vi "PmuPktDecode.vi"(8 "error in (no error)":errorcluster, 10 "PktData":string) -> (0 "error out":errorcluster, 1 "MsgVersion":u8, 2 "PMUDataType":T1, 3 "PktData":u8[](array[numeric]) format="%x", 5 "SyncOK":bool)   [LabVIEW 2014, in "SensorPlugins.lvlib" / "PmuBase.lvclass"]
uses:
  PmuBase.lvclass
  Typedef/PMUDataType.ctl
  <vilib>/Utility/error.llb/Error Cluster From Error Code.vi
  <vilib>/ErrorRing/Error Ring.xnode
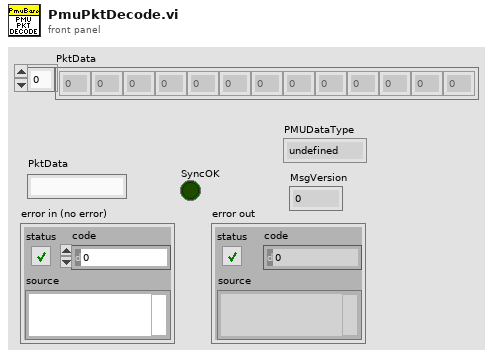
[diagram p1: front panel]
types:
  T1 = typedef "SensorPlugins.lvlib/PmuBase.lvclass/PMUDataType.ctl" = enum16{"undefined", "data", "header", "config 1", "config 2", "config 3", "command"}
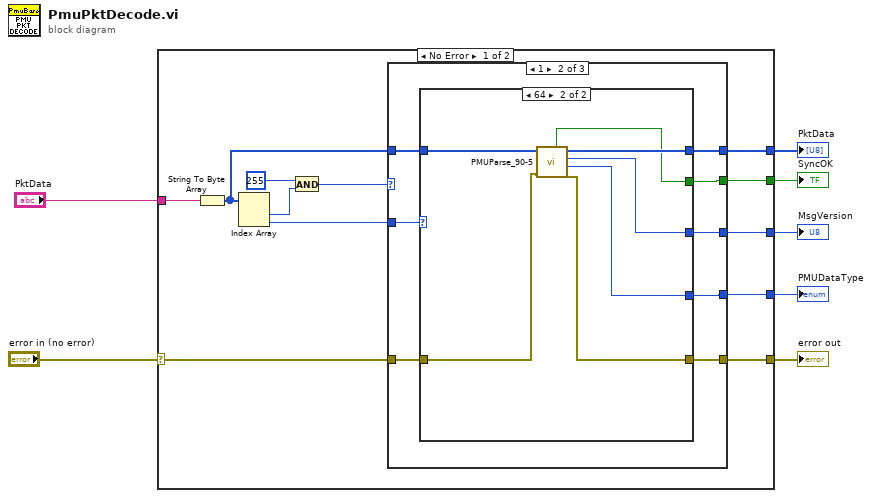
[diagram p0: block diagram]
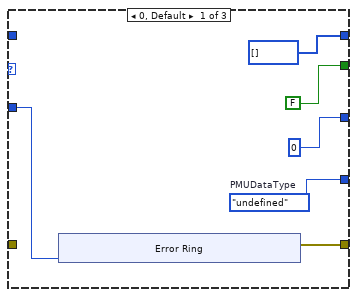
[diagram p2: hidden frame]
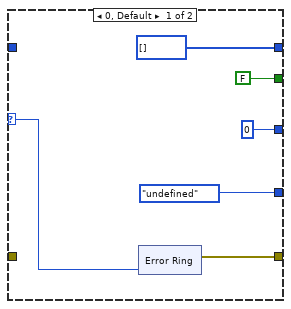
[diagram p3: hidden frame]
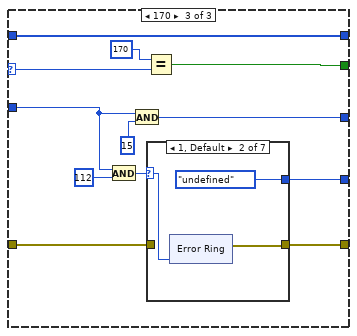
[diagram p4: hidden frame]
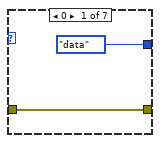
[diagram p5: hidden frame]
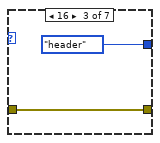
[diagram p6: hidden frame]
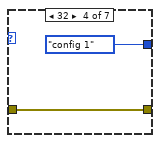
[diagram p7: hidden frame]
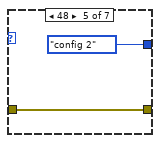
[diagram p8: hidden frame]
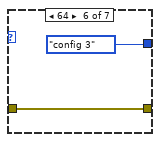
[diagram p9: hidden frame]
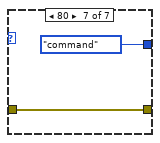
[diagram p10: hidden frame]
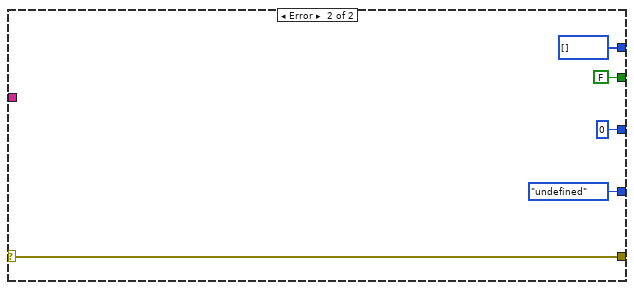
[diagram p11: hidden frame]
diagram:
  n1 = case shown="No Error" "error in (no error)" {
    selector: "error in (no error)" -> [w8 w99]
    tunnel: "PktData" -> [w17 _]
    tunnel: [w15 w99] -> w5
    tunnel: [w12 PMUDataType."undefined" ("PMUDataType")] -> w4
    tunnel: [w11 u8 0 ("MsgVersion")] -> w3
    tunnel: [w10 FALSE ("SyncOK")] -> w2
    tunnel: [w9 u8[] [] ("unsigned byte array")] -> w1
    frame No Error {
      n2 = String To Byte Array(string=w17) -> (unsigned byte array=w13:u8[])
      n3 = Index Array(array=w13) -> (element #1=w18:u8, element #2=w16:u8)  [unwired: 2 in]
      n4 = And(x=u8 255, y=w18) -> (x .and. y?=w14:u8)
      n5 = case shown="1" w14 {
        selector: w14 -> [_ _ w66]
        tunnel: [w24 w39 w62] -> w15
        tunnel: w16 -> [w25 w40 w61]
        tunnel: w13 -> [_ w34 w68]
        tunnel: [w23 w38 w64] -> w12
        tunnel: [u8 0 ("MsgVersion") w37 w65] -> w11
        tunnel: [FALSE ("SyncOK") w36 w67] -> w10
        tunnel: [u8[] [] ("PktData") w35 w68] -> w9
        tunnel: w8 -> [_ w33 w63]
        frame 0, Default {
          w23 = PMUDataType."undefined"  # PMUDataType
          n6 = xnode "Error Ring"("parameter 0"=w25) -> ("error out"=w24:errorcluster)
        }
        frame 1 {
          n7 = case shown="64" w40 {
            selector: w40 -> [w46 _]
            tunnel: [w45 w58] -> w39
            tunnel: [PMUDataType."undefined" ("PMUDataType") w54] -> w38
            tunnel: [u8 0 ("MsgVersion") w56] -> w37
            tunnel: [FALSE ("SyncOK") w55] -> w36
            tunnel: [u8[] [] ("unsigned byte array") w57] -> w35
            tunnel: w34 -> [_ w60]
            tunnel: w33 -> [_ w59]
            frame 0, Default {
              n8 = xnode "Error Ring"("parameter 0"=w46) -> ("error out"=w45:errorcluster)
            }
            frame 64 {
              n9 = call "PMUParse_90-5.vi"("error in (no error)"=w59, "DUT Data Row"=w60) -> ("error out"=w58:errorcluster, "PMUDataType"=w54:T1, "MsgVersion"=w56:u8, "PktData out"=w57:u8[], "SyncOK"=w55:bool)  [unwired: 5 in]
            }
          }
        }
        frame 170 {
          n10 = And(x=w61, y=u8 112) -> (x .and. y?=w72:u8)
          n11 = And(x=w61, y=u8 15) -> (x .and. y?=w65:u8)
          n12 = Equal?(x=u8 170, y=w66) -> (x = y?=w67:bool)
          n13 = case shown="1, Default" w72 {
            selector: w72 -> [_ w76 _ _ _ _ _]
            tunnel: [PMUDataType."data" ("PMUDataType") PMUDataType."undefined" ("PMUDataType") PMUDataType."header" ("PMUDataType") PMUDataType."config 1" ("PMUDataType") PMUDataType."config 2" ("PMUDataType") PMUDataType."config 3" ("PMUDataType") PMUDataType."command" ("PMUDataType")] -> w64
            tunnel: w63 -> [w73 _ w85 w87 w89 w91 w93]
            tunnel: [w73 w75 w85 w87 w89 w91 w93] -> w62
            frame 0 {
            }
            frame 1, Default {
              n14 = xnode "Error Ring"("parameter 0"=w76) -> ("error out"=w75:errorcluster)
            }
            frame 16 {
            }
            frame 32 {
            }
            frame 48 {
            }
            frame 64 {
            }
            frame 80 {
            }
          }
        }
      }
    }
    frame Error {
    }
  }
  "error out" <- w5
  "PktData" <- w1
  "SyncOK" <- w2
  "MsgVersion" <- w3
  "PMUDataType" <- w4
